vi "GreenRedColorMap.vi"(4 "DATA IN":u32[](array[numeric]), 5 "HWSettings":T1={"Nr. of Columns"=1, "Nr. of Rows"=18, "OverSampling"=10, "Fetch Rate "=20, "Sampling Rate"=50000, "Nr. of BNC inputs"=3, "Sample Strip Length"=10} caption="Hardware Settingss") -> (1 "percentFull":dbl, 2 "ColorOut":u32[](array[numeric]))   [LabVIEW 2012]
uses:
  controls/General Hardware config.ctl
panel:
  # "Array"
  # "Acq. System"
  # "Other analog Input"
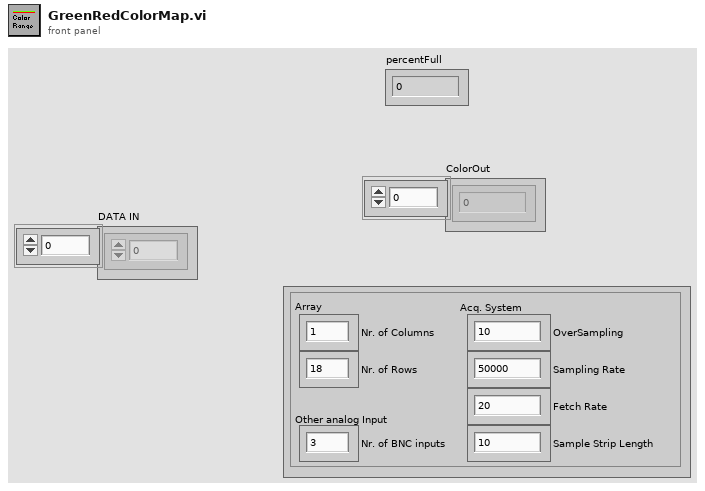
[diagram p1: front panel]
types:
  T1 = typedef "General Hardware config.ctl" = cluster{"Nr. of Columns":i32, "Nr. of Rows":i32, "OverSampling":i32, "Fetch Rate ":i32, "Sampling Rate":i32, "Nr. of BNC inputs":i32, "Sample Strip Length":i32}
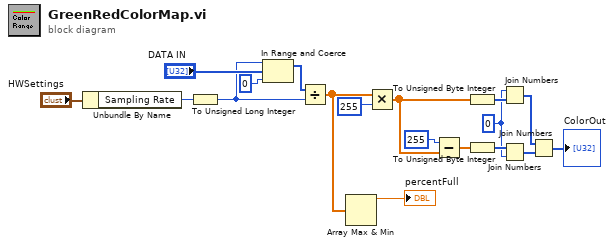
[diagram p0: block diagram]
diagram:
  w8 = i8 0 ("lo")
  n1 = Unbundle By Name("HWSettings") -> ("Sampling Rate"=w2:i32)
  n2 = To Unsigned Long Integer(number=w2) -> (unsigned 32bit integer=w1:u32)
  n3 = In Range and Coerce(upper limit=w1, x="DATA IN", lower limit=u32 0 ("Lower Limit")) -> (coerced(x)=w18:u32[])  [unwired: 1 out]
  n4 = Divide(x=w18, y=w1) -> (x/y=w6:dbl[])
  n5 = Array Max & Min(array=w6) -> (max value=→"percentFull":dbl)  [unwired: 3 out]
  n6 = Multiply(x=w6, y=255) -> (x*y=w12:dbl[])
  n7 = Subtract(x=255, y=w12) -> (x-y=w15:dbl[])
  n8 = To Unsigned Byte Integer(number=w12) -> (unsigned 8bit integer=w13:u8[])
  n9 = To Unsigned Byte Integer(number=w15) -> (unsigned 8bit integer=w14:u8[])
  n10 = Join Numbers(hi=w8, lo=w13) -> ((hi.lo)=w10:u16[])
  n11 = Join Numbers(hi=w14, lo=w8) -> ((hi.lo)=w9:u16[])
  n12 = Join Numbers(hi=w10, lo=w9) -> ((hi.lo)=→"ColorOut":u32[])
